vi "SPD.Read SPD Telemetry.vi"(8 "Error In":errorcluster, 11 "SPD.Stand Ctrl in":T1 {"spdDeviceSession"."hidSPD.Controller"."HV_bias" format="%#_6p, V"; "spdDeviceSession"."hidSPD.Controller"."TSet" format="%#_6p, DegC"}) -> (0 "Error Out":errorcluster, 1 "Diod Temprature":sgl, 2 "Heatsink Temprature":sgl, 3 "SPD.Stand Ctrl out":T1 {"spdDeviceSession"."hidSPD.Controller"."HV_bias" format="%#_6p, V"; "spdDeviceSession"."hidSPD.Controller"."TSet" format="%#_6p, DegC"}, 4 "Ready":bool)   [LabVIEW 2018]
uses:
  typedefs/SPD.Stand Ctrl.ctl
  Instruments/SPD HID Interface/hidSPDLibForLabView/LibVIs/hidSPD Controls/hidSPD Device Session.ctl
  Instruments/SPD HID Interface/hidSPDLibForLabView/LibVIs/hidSPD Controls/hidSPD Controller.ctl
  Instruments/KC705 DevBoard/typedefs/DevB.Session.ctl
  Instruments/KeySight 53230A/typedefs/FreqC.Session.ctl
  Instruments/KeySight 8164B/KeySight 8164B LAN InstrLib/typedefs/KeySight 8164B control.ctl
  Instruments/LeCroy SDA830/typedefs/LeCroy.Session.ctl
  typedefs/SPD.Events.ctl
  <vilib>/Utility/config.llb/Config Data RefNum.ctl
  typedefs/SPD.Meas Result.ctl
  Instruments/SPD HID Interface/hidSPDLibForLabView/LibVIs/hidSPD Read Report/hidSPD Read Telemetry.vi
  Instruments/SPD HID Interface/hidSPDLibForLabView/hidSPDLibForLabView.lvlib
  Instruments/KeySight 8164B/KeySight 8164B LAN InstrLib.lvlib
  <vilib>/Utility/config.llb/NI_LVConfig.lvlib
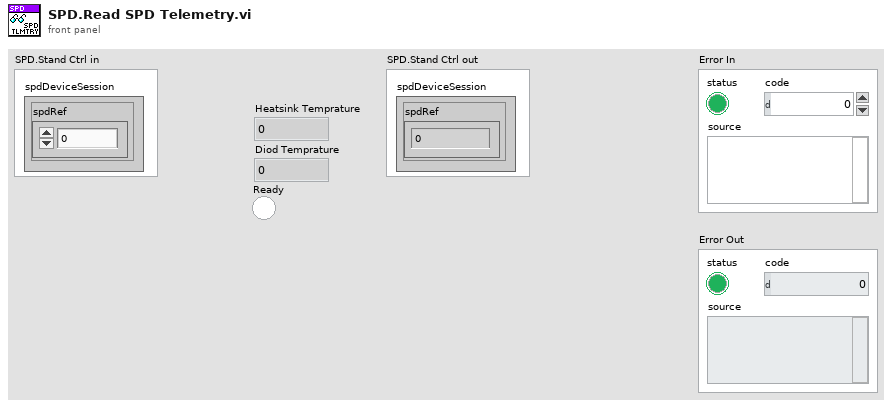
[diagram p1: front panel]
types:
  T1 = typedef "SPD.Stand Ctrl.ctl" = cluster{"spdDeviceSession":T2, "DevBSession":T4, "FreqCSession":T5, "8164BSession":T6, "LeCroySession":T7, "Events":T8, "configFile":T9, "SPD.Result":T10}
  T2 = typedef "hidSPDLibForLabView.lvlib/hidSPD Device Session.ctl" = cluster{"spdRef":u64, "connected":bool, "spdName":string, "hidSPD.Controller":T3}
  T3 = typedef "hidSPDLibForLabView.lvlib/hidSPD Controller.ctl" = cluster{"TSet":sgl, "HV_bias":sgl, "DDS_stb_code":u16}
  T4 = typedef "DevB.Session.ctl" = cluster{"DevBRef":refnum<visa-resource-name>, "connected":bool}
  T5 = typedef "FreqC.Session.ctl" = cluster{"FreqCRef":refnum<visa-resource-name>, "timeout":dbl, "Gate":dbl, "connected":bool}
  T6 = typedef "KeySight 8164B LAN InstrLib.lvlib/KeySight 8164B control.ctl" = cluster{"Connection ID":refnum<k5>, "Connected":bool, "Info":string, "Slots Info":string[]}
  T7 = typedef "LeCroy.Session.ctl" = cluster{"LeCroySession":refnum<visa-resource-name>, "connected":bool}
  T8 = typedef "SPD.Events.ctl" = cluster{"DCRTest":refnum<user-event>, "Stop":refnum<user-event>}
  T9 = typedef "NI_LVConfig.lvlib/Config Data RefNum.ctl" = refnum<k1>
  T10 = typedef "SPD.Meas Result.ctl" = cluster{"HV_Bias":dbl[][][], "Stb_code":dbl[], "Temprature":dbl[], "Data":dbl[][][][]}
  T11 = typedef "hidSPDLibForLabView.lvlib/hidSPD Simple Report.ctl" = cluster{"Heatsink Temprature":sgl, "Diod Temprature":sgl, "TEC-voltage":sgl, "Diod Bias":sgl, "RF Power":sgl, "Thrm_used":sgl, "Thrm_end":sgl, "Thrm_error":sgl, "stableI":sgl, "pid_error":sgl, "strobe code used":u16, "SPD number":u8, "SPD ready":u8, "status SPD":u32}
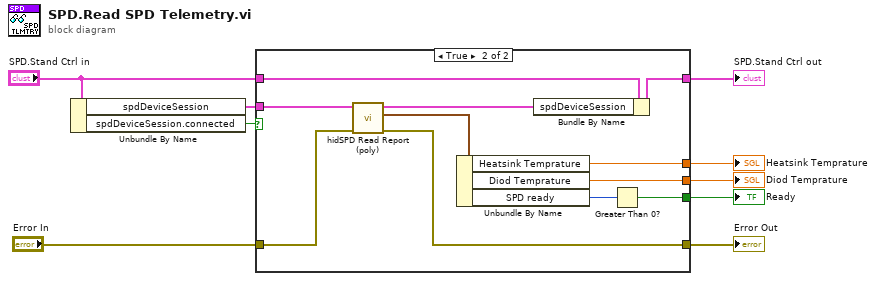
[diagram p0: block diagram]
diagram:
  n1 = Unbundle By Name("SPD.Stand Ctrl in") -> ("spdDeviceSession"=w9:T2, "spdDeviceSession.connected"=w1:bool)
  n2 = case shown="True" w1 {
    tunnel: w9 -> [_ w22]
    tunnel: "Error In" -> [w10 w21]
    tunnel: "SPD.Stand Ctrl in" -> [w11 w20]
    tunnel: [w11 w19] -> w6
    tunnel: [w10 w16] -> w5
    tunnel: [_ w15] -> w4
    tunnel: [_ w14] -> w3
    tunnel: [_ w12] -> w2
    frame False {
    }
    frame True {
      n3 = call-poly "hidSPD Read Report (poly).vi"("error in (no error)"=w21, "spdDevSession in"=w22) -> ("error out"=w16:errorcluster, "telemetry"=w17:T11, "spdDevSession out"=w18:T2)  [unwired: 7 in]
      n4 = Unbundle By Name(w17) -> ("Heatsink Temprature"=w15:sgl, "Diod Temprature"=w14:sgl, "SPD ready"=w13:u8)
      n5 = Bundle By Name(cluster=w20, "spdDeviceSession"=w18) -> (w19:T1)
      n6 = Greater Than 0?(x=w13) -> (x > 0?=w12:bool)
    }
  }
  "SPD.Stand Ctrl out" <- w6
  "Error Out" <- w5
  "Heatsink Temprature" <- w4
  "Diod Temprature" <- w3
  "Ready" <- w2
